vi "Write Graph-Chart Cursor Names.vi"(8 "error in":errorcluster, 10 "Value":string[](array[string]), 11 "Graph / Chart Reference in":refnum<vi>) -> (0 "error out":errorcluster, 3 "Graph / Chart Reference out":refnum<vi>)   [LabVIEW 2020, in "G-Unicode.lvlib"]
uses:
  G-Unicode.lvlib
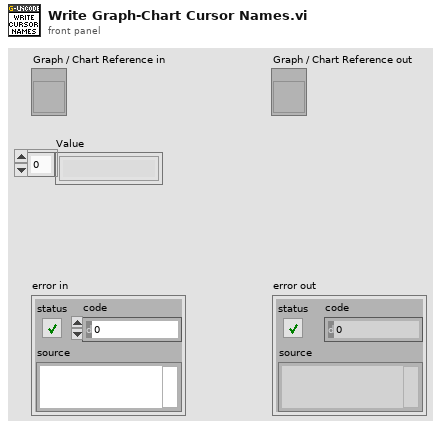
[diagram p1: front panel]
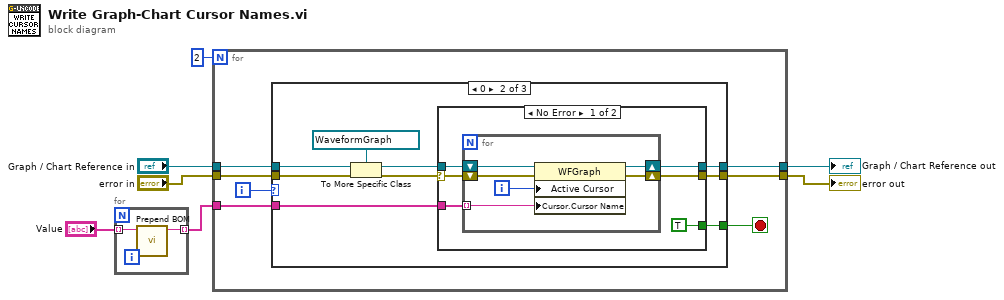
[diagram p0: block diagram]
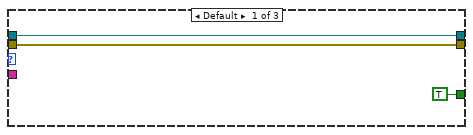
[diagram p2: hidden frame]
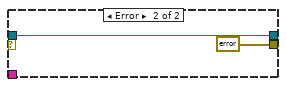
[diagram p3: hidden frame]
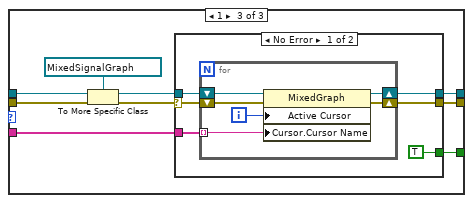
[diagram p4: hidden frame]
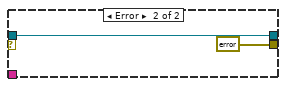
[diagram p5: hidden frame]
diagram:
  n1 = for {
    tunnel: "Value" -> [w9] mode=indexing
    tunnel: [w8] -> w1 mode=indexing
    n2 = call "Prepend BOM.vi"("String"=w9) -> ("String with BOM"=w8:string)  [unwired: 9 in, 1 out]
  }
  n3 = for {
    N: 2 -> [_]
    tunnel: "error in" -> [w16]
    tunnel: [w15] -> w6
    tunnel: [w14] -> w5
    tunnel: "Graph / Chart Reference in" -> [w13]
    tunnel: w1 -> [w12]
    i -> [w11]
    stop <- w10 stop-if-true
    n4 = case shown="0" w11 {
      tunnel: w16 -> [w18 w23 w46]
      tunnel: [w19 w28 w51] -> w15
      tunnel: [w18 w27 w50] -> w14
      tunnel: w13 -> [w19 w26 w49]
      tunnel: w12 -> [_ w25 w48]
      tunnel: [TRUE w20 w43] -> w10
      frame Default {
      }
      frame 0 {
        n5 = To More Specific Class(target class=refnum<vi> refnum ("Graph / Chart Reference in"), reference=w26, error in=w23) -> (specific class reference=w24:refnum<vi>, error out=w21:errorcluster)
        n6 = case shown="No Error" w21 {
          selector: w21 -> [w30 _]
          tunnel: [w34 w41] -> w28
          tunnel: [w33 errorcluster {"status"=FALSE, "code"=0, "source"=""} ("error IO")] -> w27
          tunnel: w25 -> [w32 _]
          tunnel: w24 -> [w31 w41]
          tunnel: [TRUE _] -> w20
          frame No Error {
            n7 = for {
              tunnel: w32 -> [w36] mode=indexing
              shift-right: [w38] -> w33
              shift-left: w30 -> [w40]
              shift-right: [w39] -> w34
              shift-left: w31 -> [w37]
              i -> [w35]
              n8 = property class="WFGraph"(reference=w37, error in=w40, "Active Cursor"=w35, "Cursor.Cursor Name"=w36) -> (reference out=w39:refnum<vi>, error out=w38:errorcluster)
            }
          }
          frame Error {
          }
        }
      }
      frame 1 {
        n9 = To More Specific Class(target class=refnum<vi> refnum ("Graph / Chart Reference in"), reference=w49, error in=w46) -> (specific class reference=w47:refnum<vi>, error out=w44:errorcluster)
        n10 = case shown="No Error" w44 {
          selector: w44 -> [w53 _]
          tunnel: [w57 w64] -> w51
          tunnel: [w56 errorcluster {"status"=FALSE, "code"=0, "source"=""} ("error IO")] -> w50
          tunnel: w48 -> [w55 _]
          tunnel: w47 -> [w54 w64]
          tunnel: [TRUE _] -> w43
          frame No Error {
            n11 = for {
              tunnel: w55 -> [w59] mode=indexing
              shift-right: [w61] -> w56
              shift-left: w53 -> [w63]
              shift-right: [w62] -> w57
              shift-left: w54 -> [w60]
              i -> [w58]
              n12 = property class="MixedGraph"(reference=w60, error in=w63, "Active Cursor"=w58, "Cursor.Cursor Name"=w59) -> (reference out=w62:refnum<vi>, error out=w61:errorcluster)
            }
          }
          frame Error {
          }
        }
      }
    }
  }
  "error out" <- w5
  "Graph / Chart Reference out" <- w6
